vi "UDP config.vi"(8 "error in":errorcluster, 9 "par 3":T1={"Loop time"={"Period [ms]"=5, "Processor"=-2}, "COM"={"COM IP"="192.168.8.70", "COM port"=30005, "Local port"=5556, "Next_IP 1"=0, "Next_IP 2"=0, "Next_IP 3"=0, "Next_IP 4"=0}, "O2Sensor1"={"Lambda"={"LSU4.2 Lambda"=[], "LSU4.2 Ip"=[], "LSU4.9 Lambda"=[], "LSU4.9 Ip"=[], "LZA03 Lambda"=[], "LZA03 Ip"=[], "LZA08 Lambda"=[], "LZA08 Ip"=[], "Custom Lambda"=[], "Custom Ip"=[]}, "Temp"={"LSU4.2 Temp"=[], "LSU4.2 Ohm"=[], "LSU4.9 Temp"=[], "LSU4.9 Ohm"=[], "LZA03 Temp"=[], "LZA03 Ohm"=[], "LZA08 Temp"=[], "LZA08 Ohm"=[], "Custom Temp"=[], "Custom Ohm"=[]}, "Lambda Type"=enum."LSU4.2", "PID"={"Ki"=0.0, "Kp"=0.0, "Kd"=0.0, "FeedFW"=0.0}}, "O2Sensor2"={"Lambda"={"LSU4.2 Lambda"=[], "LSU4.2 Ip"=[], "LSU4.9 Lambda"=[], "LSU4.9 Ip"=[], "LZA03 Lambda"=[], "LZA03 Ip"=[], "LZA08 Lambda"=[], "LZA08 Ip"=[], "Custom Lambda"=[], "Custom Ip"=[]}, "Temp"={"LSU4.2 Temp"=[], "LSU4.2 Ohm"=[], "LSU4.9 Temp"=[], "LSU4.9 Ohm"=[], "LZA03 Temp"=[], "LZA03 Ohm"=[], "LZA08 Temp"=[], "LZA08 Ohm"=[], "Custom Temp"=[], "Custom Ohm"=[]}, "Lambda Type"=enum."LSU4.2", "PID"={"Ki"=0.0, "Kp"=0.0, "Kd"=0.0, "FeedFW"=0.0}}, "O2Sensor3"={"Lambda"={"LSU4.2 Lambda"=[], "LSU4.2 Ip"=[], "LSU4.9 Lambda"=[], "LSU4.9 Ip"=[], "LZA03 Lambda"=[], "LZA03 Ip"=[], "LZA08 Lambda"=[], "LZA08 Ip"=[], "Custom Lambda"=[], "Custom Ip"=[]}, "Temp"={"LSU4.2 Temp"=[], "LSU4.2 Ohm"=[], "LSU4.9 Temp"=[], "LSU4.9 Ohm"=[], "LZA03 Temp"=[], "LZA03 Ohm"=[], "LZA08 Temp"=[], "LZA08 Ohm"=[], "Custom Temp"=[], "Custom Ohm"=[]}, "Lambda Type"=enum."LSU4.2", "PID"={"Ki"=0.0, "Kp"=0.0, "Kd"=0.0, "FeedFW"=0.0}}, "O2Sensor4"={"Lambda"={"LSU4.2 Lambda"=[], "LSU4.2 Ip"=[], "LSU4.9 Lambda"=[], "LSU4.9 Ip"=[], "LZA03 Lambda"=[], "LZA03 Ip"=[], "LZA08 Lambda"=[], "LZA08 Ip"=[], "Custom Lambda"=[], "Custom Ip"=[]}, "Temp"={"LSU4.2 Temp"=[], "LSU4.2 Ohm"=[], "LSU4.9 Temp"=[], "LSU4.9 Ohm"=[], "LZA03 Temp"=[], "LZA03 Ohm"=[], "LZA08 Temp"=[], "LZA08 Ohm"=[], "Custom Temp"=[], "Custom Ohm"=[]}, "Lambda Type"=enum."LSU4.2", "PID"={"Ki"=0.0, "Kp"=0.0, "Kd"=0.0, "FeedFW"=0.0}}, "#ch_choise"=enum."O2Sim_2ch", "Mode"=enum."SLSC Mode"}, 10 "Cluster in":T3, 11 "Data In":dbl[](array[numeric])) -> (0 "error out":errorcluster, 2 "connection error?":bool, 3 "Cluster out":T3)   [LabVIEW 2017]
uses:
  Par.ctl
  LambdaType.ctl
panel:
  in  "errors to clear":i32[](array[ring])=[1, 56, 60, 62, 63, 64, 66] items=["No Error", "Argument Error", "Memory Full", "Out of Zone", "End of File", "File Already Open", "Generic File IO Error", "File Not Found", "File Permission Error", "Disk Full", "Duplicate Path", "Too Many Files Open", "Not Enabled", "Resource File Not Found", "Cannot Add Resource", "Resource Not Found", "Image Not Found", "Image Memory Error", "Pen Does Not Exist", "Config Bad Type", "Config Token Not Found", "Config Parse Error", "Config Memory Error", "Bad External Code Format", "Bad External Code Offset", "External Code Not Present", "Null Window", "Destroy Window Mixup", "Null Menu", "Print Aborted", "Bad Print Record", "Print Driver Error", "Windows Error During Print", "Memory Error During Print", "Print Dialog Error", "Generic Print Error", "Invalid Device Refnum", "Device Not Found", "Device Parameter Error", "Device Unit Error", "Can't Open Device", "Device Call Aborted", "Generic Error", "Cancelled By User", "Object ID Too Low", "Object ID Too High", "Object Not In Heap", "Unknown Heap", "Bad DefProc ID", "DefProc Not In Table", "Message Out Of Range", "Null Method", "Unknown Message", "Manager Call Not Supported", "Bad address", "Connection In progress", "Connection timed out", "Connection is already in progress", "Network attribute not supported", "Network error", "Address in use", "System out of memory", "Connection aborted", "Connection refused", "Connection is not connected", "Connection is already connected", "Connection closed", "Initialize error (interapplication manager)", "Bad occurrence", "Wait on unbound occurrence handler", "Occurrence queue overflow", "Bad path", "Semaphore not signaled", "Unrecognized type (interapplication manager)"]
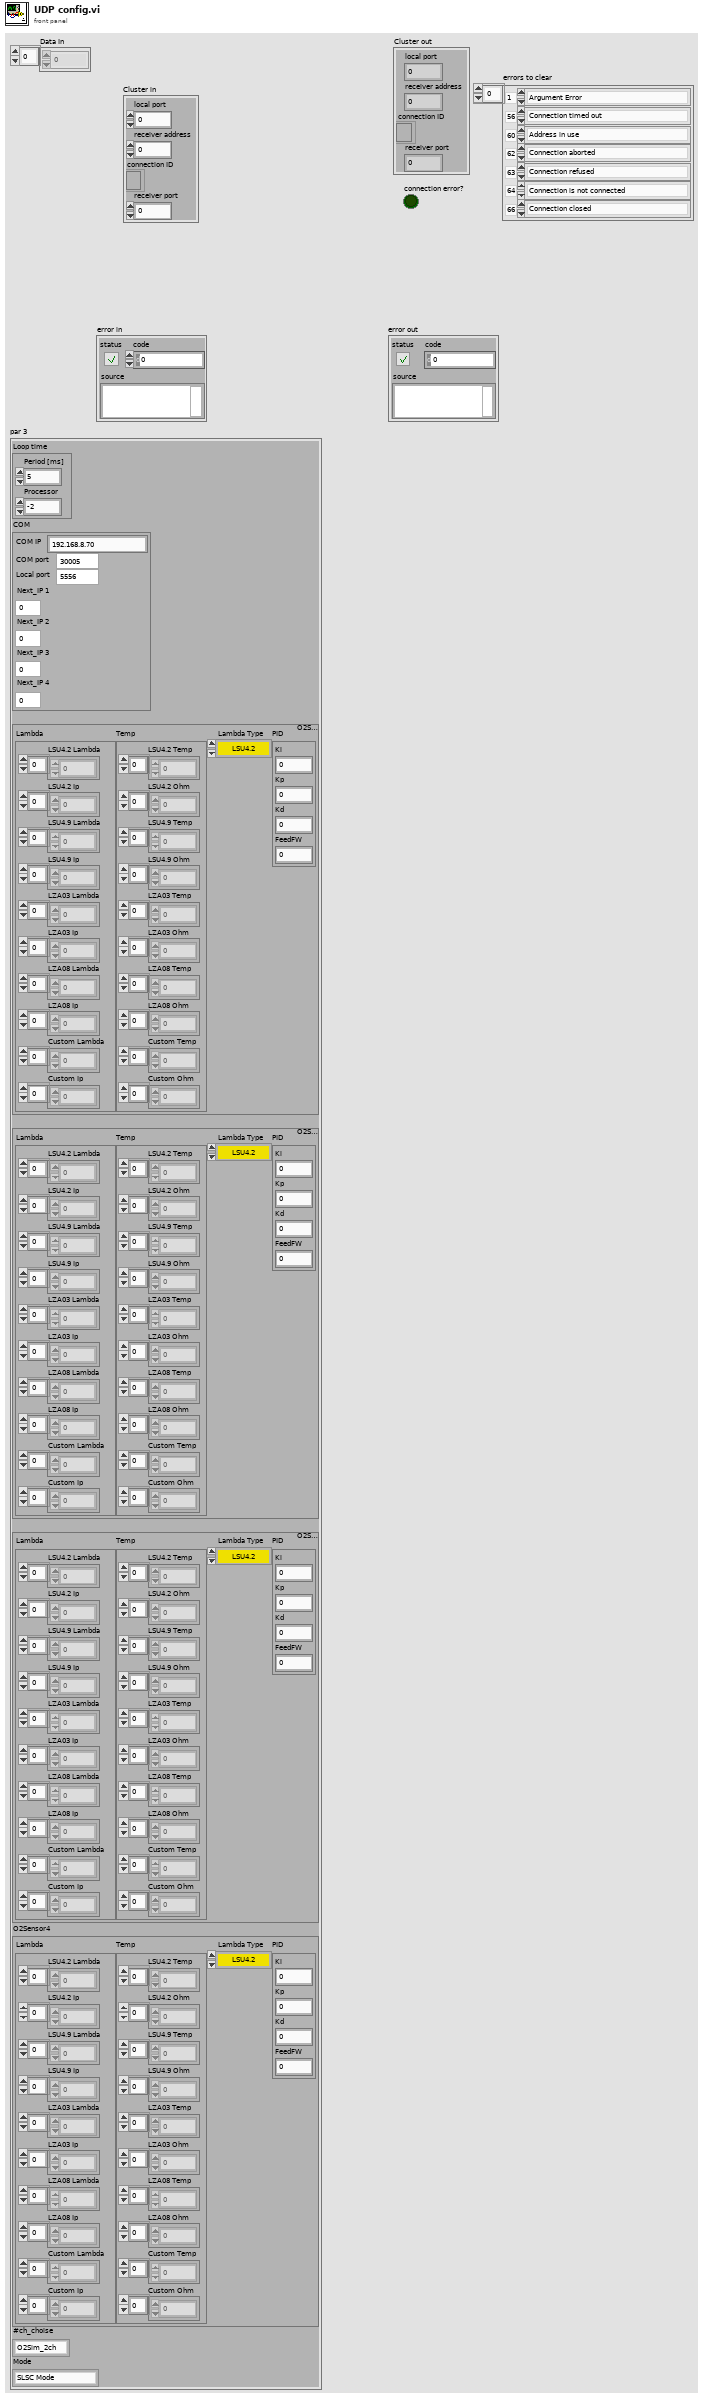
[diagram p1: front panel]
types:
  T1 = typedef "Par.ctl" = cluster{"Loop time":cluster{"Period [ms]":i64, "Processor":i32}, "COM":cluster{"COM IP":string, "COM port":u64, "Local port":u64, "Next_IP 1":u32, "Next_IP 2":u32, "Next_IP 3":u32, "Next_IP 4":u32}, "O2Sensor1":cluster{"Lambda":cluster{"LSU4.2 Lambda":dbl[], "LSU4.2 Ip":dbl[], "LSU4.9 Lambda":dbl[], "LSU4.9 Ip":dbl[], "LZA03 Lambda":dbl[], "LZA03 Ip":dbl[], "LZA08 Lambda":dbl[], "LZA08 Ip":dbl[], "Custom Lambda":dbl[], "Custom Ip":dbl[]}, "Temp":cluster{"LSU4.2 Temp":dbl[], "LSU4.2 Ohm":dbl[], "LSU4.9 Temp":dbl[], "LSU4.9 Ohm":dbl[], "LZA03 Temp":dbl[], "LZA03 Ohm":dbl[], "LZA08 Temp":dbl[], "LZA08 Ohm":dbl[], "Custom Temp":dbl[], "Custom Ohm":dbl[]}, "Lambda Type":T2, "PID":cluster{"Ki":dbl, "Kp":dbl, "Kd":dbl, "FeedFW":dbl}}, "O2Sensor2":cluster{"Lambda":cluster{"LSU4.2 Lambda":dbl[], "LSU4.2 Ip":dbl[], "LSU4.9 Lambda":dbl[], "LSU4.9 Ip":dbl[], "LZA03 Lambda":dbl[], "LZA03 Ip":dbl[], "LZA08 Lambda":dbl[], "LZA08 Ip":dbl[], "Custom Lambda":dbl[], "Custom Ip":dbl[]}, "Temp":cluster{"LSU4.2 Temp":dbl[], "LSU4.2 Ohm":dbl[], "LSU4.9 Temp":dbl[], "LSU4.9 Ohm":dbl[], "LZA03 Temp":dbl[], "LZA03 Ohm":dbl[], "LZA08 Temp":dbl[], "LZA08 Ohm":dbl[], "Custom Temp":dbl[], "Custom Ohm":dbl[]}, "Lambda Type":T2, "PID":cluster{"Ki":dbl, "Kp":dbl, "Kd":dbl, "FeedFW":dbl}}, "O2Sensor3":cluster{"Lambda":cluster{"LSU4.2 Lambda":dbl[], "LSU4.2 Ip":dbl[], "LSU4.9 Lambda":dbl[], "LSU4.9 Ip":dbl[], "LZA03 Lambda":dbl[], "LZA03 Ip":dbl[], "LZA08 Lambda":dbl[], "LZA08 Ip":dbl[], "Custom Lambda":dbl[], "Custom Ip":dbl[]}, "Temp":cluster{"LSU4.2 Temp":dbl[], "LSU4.2 Ohm":dbl[], "LSU4.9 Temp":dbl[], "LSU4.9 Ohm":dbl[], "LZA03 Temp":dbl[], "LZA03 Ohm":dbl[], "LZA08 Temp":dbl[], "LZA08 Ohm":dbl[], "Custom Temp":dbl[], "Custom Ohm":dbl[]}, "Lambda Type":T2, "PID":cluster{"Ki":dbl, "Kp":dbl, "Kd":dbl, "FeedFW":dbl}}, "O2Sensor4":cluster{"Lambda":cluster{"LSU4.2 Lambda":dbl[], "LSU4.2 Ip":dbl[], "LSU4.9 Lambda":dbl[], "LSU4.9 Ip":dbl[], "LZA03 Lambda":dbl[], "LZA03 Ip":dbl[], "LZA08 Lambda":dbl[], "LZA08 Ip":dbl[], "Custom Lambda":dbl[], "Custom Ip":dbl[]}, "Temp":cluster{"LSU4.2 Temp":dbl[], "LSU4.2 Ohm":dbl[], "LSU4.9 Temp":dbl[], "LSU4.9 Ohm":dbl[], "LZA03 Temp":dbl[], "LZA03 Ohm":dbl[], "LZA08 Temp":dbl[], "LZA08 Ohm":dbl[], "Custom Temp":dbl[], "Custom Ohm":dbl[]}, "Lambda Type":T2, "PID":cluster{"Ki":dbl, "Kp":dbl, "Kd":dbl, "FeedFW":dbl}}, "#ch_choise":enum16{"O2Sim_2ch", "O2Sim_4ch"}, "Mode":enum16{"SLSC Mode", "ANALOG Mode"}}
  T2 = typedef "LambdaType.ctl" = enum16{"LSU4.2", "LSU4.9", "LZA03", "LZA08", "Custom", "[mA]"}
  T3 = cluster{"local port":u16, "receiver address":u32, "connection ID":refnum<k16>, "receiver port":u16}
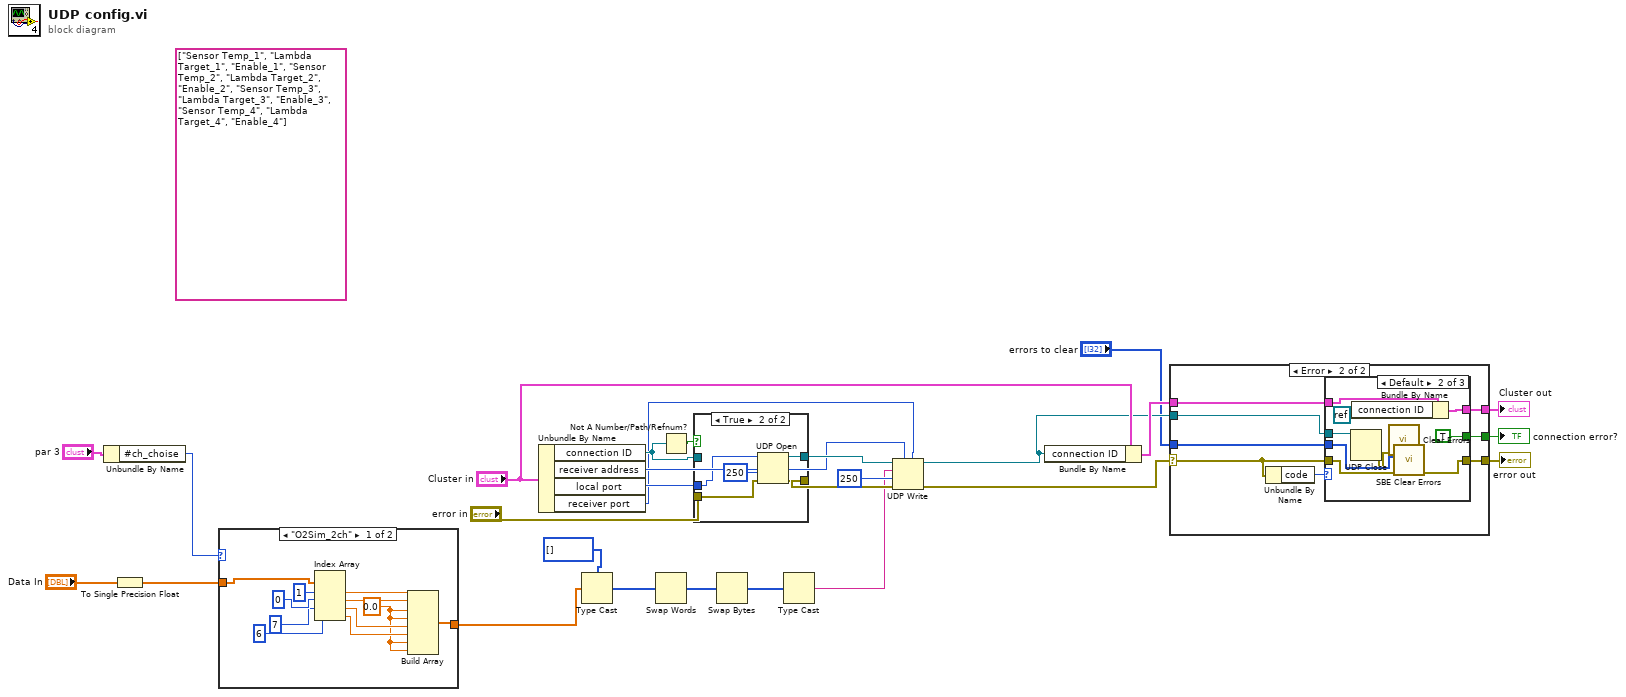
[diagram p0: block diagram]
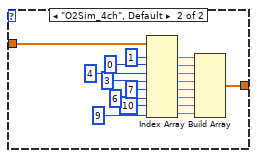
[diagram p2: hidden frame]
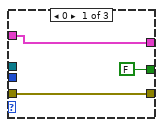
[diagram p4: hidden frame]
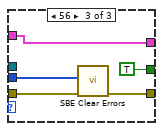
[diagram p5: hidden frame]
diagram:
  (unwired) string[] ["Sensor Temp_1", "Lambda Target_1", "Enable_1", "Sensor Temp_2", "Lambda Target_2", "Enable_2", "Sensor Temp_3", "Lambda Target_3", "Enable_3", "Sensor Temp_4", "Lambda Target_4", "Enable_4"] ("O2SensoSim Setpoint 2")
  n1 = Unbundle By Name("par 3") -> ("#ch_choise"=w1:enum16{"O2Sim_2ch", "O2Sim_4ch"})
  n2 = To Single Precision Float(number="Data In") -> (single precision float=w3:sgl[])
  n3 = case shown="\"O2Sim_2ch\"" w1 {
    tunnel: [w28 w40] -> w4
    tunnel: w3 -> [w32 w39]
    frame "O2Sim_2ch" {
      w29 = sgl 0.0 ("element")
      n4 = Index Array(array=w32, index #1=1 ("index"), index #2=0 ("index"), index #3=7 ("index"), index #4=6 ("index")) -> (element #1=w37:sgl, element #2=w38:sgl, element #3=w31:sgl, element #4=w30:sgl)
      n5 = Build Array(w37, w38, w29, w29, w31, w30, w29, w29) -> (w28:sgl[])
    }
    frame "O2Sim_4ch", Default {
      n6 = Index Array(array=w39, index #1=1 ("index"), index #2=0 ("index"), index #3=4 ("index"), index #4=3 ("index"), index #5=7 ("index"), index #6=6 ("index"), index #7=10 ("index"), index #8=9 ("index")) -> (element #1=w48:sgl, element #2=w47:sgl, element #3=w46:sgl, element #4=w45:sgl, element #5=w44:sgl, element #6=w43:sgl, element #7=w42:sgl, element #8=w41:sgl)
      n7 = Build Array(w48, w47, w46, w45, w44, w43, w42, w41) -> (w40:sgl[])
    }
  }
  n8 = Unbundle By Name("Cluster in") -> ("connection ID"=w26:refnum<k16>, "receiver address"=w21:u32, "local port"=w25:u16, "receiver port"=w7:u16)
  n9 = Type Cast(type=u32[] [] ("appended array"), x=w4) -> (*(type *) &x=w9:u32[])
  n10 = Swap Words(1:w9) -> (0:w10:u32[])
  n11 = Not A Number/Path/Refnum?(number/path/refnum=w26) -> (NaN/Path/Refnum?=w27:bool)
  n12 = case shown="True" w27 {
    tunnel: "error in" -> [w58 w63]
    tunnel: w26 -> [w57 _]
    tunnel: w25 -> [_ w59]
    tunnel: [w58 w62] -> w24
    tunnel: [w57 w60] -> w23
    frame False {
    }
    frame True {
      n13 = UDP Open(8:w63, 9:250 ("timeout ms (25000)"), 11:w59) -> (port=w60:refnum<k16>, 0:w62:errorcluster)  [unwired: 3 out]
    }
  }
  n14 = Swap Bytes(anything=w10) -> (byte swapped=w8:u32[])
  n15 = Type Cast(x=w8) -> (*(type *) &x=w12:string)  [unwired: 1 in]
  n16 = UDP Write(address=w21, port or service name=w7, connection ID=w23, data in=w12, 8:w24, 9:250 ("timeout ms (25000)")) -> (error out=w6:errorcluster, 3:w18:refnum<k16>)
  n17 = Bundle By Name(cluster="Cluster in", "connection ID"=w18) -> (w22:T3)
  n18 = case shown="Error" w6 {
    selector: w6 -> [w65 w71]
    tunnel: [w65 w72] -> w15
    tunnel: [_ w70] -> w16
    tunnel: "errors to clear" -> [_ w69]
    tunnel: w18 -> [_ w68]
    tunnel: w22 -> [w64 w67]
    tunnel: [w64 w66] -> w17
    frame No Error {
    }
    frame Error {
      n19 = Unbundle By Name(w71) -> ("code"=w73:i32)
      n20 = case shown="Default" w73 {
        tunnel: w71 -> [w76 w84 w89]
        tunnel: [w76 w83 w88] -> w72
        tunnel: [FALSE ("connection error?") TRUE ("connection error?") TRUE ("connection error?")] -> w70
        tunnel: w69 -> [_ w82 w87]
        tunnel: w68 -> [_ w81 _]
        tunnel: w67 -> [w74 w80 w86]
        tunnel: [w74 w79 w86] -> w66
        frame 0 {
        }
        frame Default {
          n21 = UDP Close(connection ID=w81) -> (error out=w77:errorcluster)  [unwired: 1 in, 1 out]
          n22 = Bundle By Name(cluster=w80, "connection ID"=refnum<k0> refnum) -> (w79:T3)
          n23 = call <vilib>:"Clear Errors.vi"("error in (no error)"=w77) -> ()  [unwired: 5 in, 2 out]
          n24 = call "SBE Clear Errors.vi"("error in (no error)"=w84, "Error Codes Array"=w82) -> ("error out"=w83:errorcluster)  [unwired: 8 in, 1 out]
        }
        frame 56 {
          n25 = call "SBE Clear Errors.vi"("error in (no error)"=w89, "Error Codes Array"=w87) -> ("error out"=w88:errorcluster)  [unwired: 8 in, 1 out]
        }
      }
    }
  }
  "Cluster out" <- w17
  "connection error?" <- w16
  "error out" <- w15
